vi "resetOutput.vi"(8 "error in (no error)":errorcluster, 11 "K2602 in":refnum<class "K2602.lvclass">) -> (0 "error out":errorcluster, 3 "K2602 out":refnum<class "K2602.lvclass">)   [LabVIEW 2009, in "Hardware.lvlib" / "Channels.lvlib" / "K2602.lvclass"]
uses:
  K2602.lvclass
  K2602.lvclass/K2602.ctl
  AnalogOutput.lvclass
  <instrlib>/Keithley 2600 Series/Keithley 2600 Series.lvlib
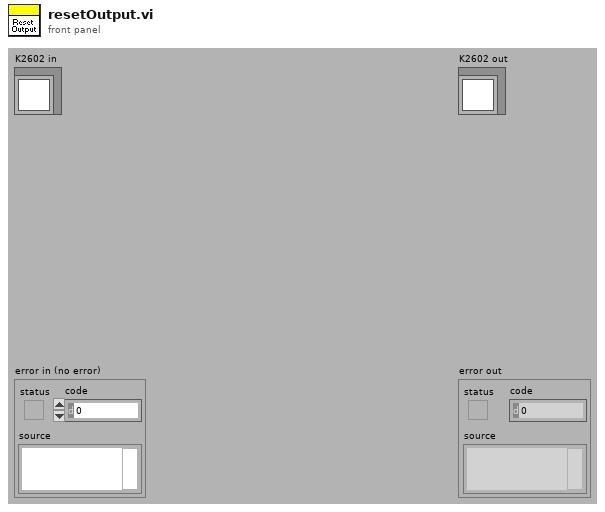
[diagram p1: front panel]
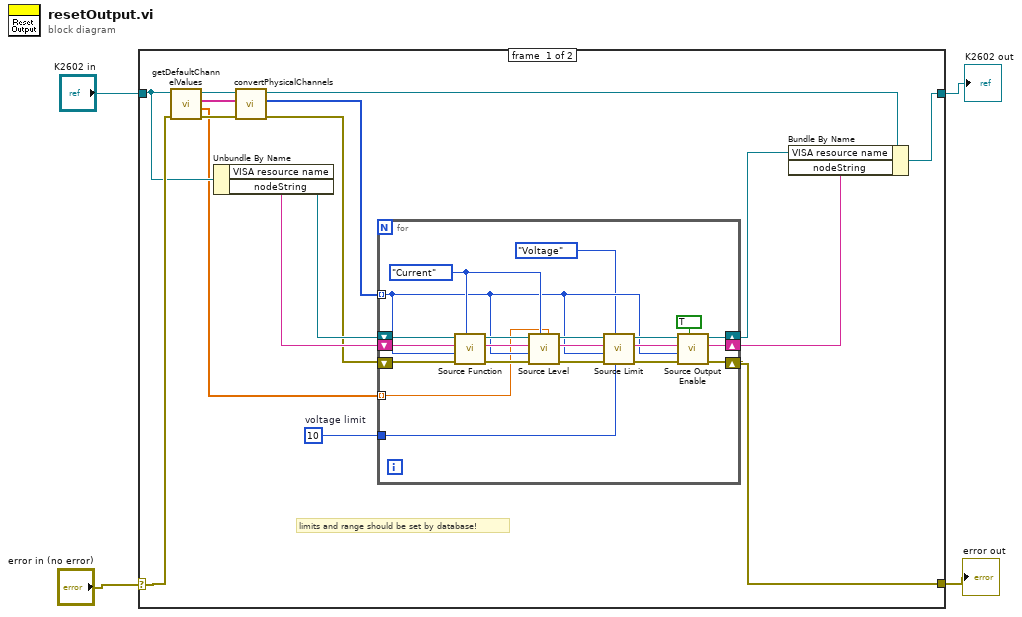
[diagram p0: block diagram]
diagram:
  n1 = case shown="No Error" "error in (no error)" {
    selector: "error in (no error)" -> [w20 w42]
    tunnel: [w6 w43] -> w4
    tunnel: "K2602 in" -> [w16 w43]
    tunnel: [w5 w42] -> w1
    frame #0 {
      w11 = 10  # voltage limit
      # "limits and range should be set by database!"
      n2 = call "getDefaultChannelValues.vi"("error in (no error)"=w20, "AnalogOutput in"=w16) -> ("error out"=w17:errorcluster, "calibratedValues"=w10:dbl[], "channel_addresses"=w18:string[], "AnalogOutput out"=w19:refnum<class "K2602.lvclass">)  [unwired: 6 in]
      n3 = Unbundle By Name(w16) -> ("VISA resource name"=w15:refnum<visa-resource-name>, "nodeString"=w14:string)
      n4 = call "convertPhysicalChannels.vi"("error in (no error)"=w17, "physicalChannels"=w18, "K2602 in"=w19) -> ("error out"=w13:errorcluster, "channel"=w12:i32[], "K2602 out"=w9:refnum<class "K2602.lvclass">)  [unwired: 6 in]
      n5 = for {
        tunnel: w12 -> [w27] mode=indexing
        tunnel: w11 -> [w25]
        tunnel: w10 -> [w24] mode=indexing
        shift-right: [w23] -> w8
        shift-left: w15 -> [w30]
        shift-right: [w22] -> w7
        shift-left: w14 -> [w29]
        shift-right: [w21] -> w5
        shift-left: w13 -> [w28]
        w31 = enum32{"Current", "Voltage"}."Current" ("Source Function (Current)")
        n6 = call <instrlib>:"Source Function.vi"("Function (Current)"=w31, "error in (no error)"=w28, "Channel (Channel A)"=w27, "Node In"=w29, "VISA resource name"=w30) -> ("error out"=w39:errorcluster, "Node Out"=w41:string, "VISA resource name out"=w40:refnum<visa-resource-name>)  [unwired: 4 out]
        n7 = call <instrlib>:"Source Level.vi"("Level (0.000)"=w24, "Function (Current)"=w31, "error in (no error)"=w39, "Channel (Channel A)"=w27, "Node In"=w41, "VISA resource name"=w40) -> ("error out"=w38:errorcluster, "Node Out"=w33:string, "VISA resource name out"=w37:refnum<visa-resource-name>)  [unwired: 3 out]
        n8 = call <instrlib>:"Source Limit.vi"("Limit (0.000)"=w25, "Function (Current)"=enum32{"Current", "Voltage"}."Voltage" ("x"), "error in (no error)"=w38, "Channel (Channel A)"=w27, "Node In"=w33, "VISA resource name"=w37) -> ("error out"=w35:errorcluster, "Node Out"=w32:string, "VISA resource name out"=w36:refnum<visa-resource-name>)  [unwired: 3 out]
        n9 = call <instrlib>:"Source Output Enable.vi"("Output (Off)"=TRUE, "error in (no error)"=w35, "Channel (Channel A)"=w27, "Node In"=w32, "VISA resource name"=w36) -> ("error out"=w21:errorcluster, "Node Out"=w22:string, "VISA resource name out"=w23:refnum<visa-resource-name>)  [unwired: 4 out]
      }
      n10 = Bundle By Name(cluster=w9, "VISA resource name"=w8, "nodeString"=w7) -> (w6:refnum<class "K2602.lvclass">)
    }
    frame #1 {
    }
  }
  "error out" <- w1
  "K2602 out" <- w4
